vi "Main.vi"(10 "VISA resource name":refnum<visa-resource-name>="COM11", 11 "Module Admin":refnum<class "Delacor_lib_QMH_Module Admin.lvclass">) -> ()   [LabVIEW 2018, in "MB switches Module.lvlib"]
doc: "This template is based off of the Queued Message Handler design pattern and the Queued Message Handler project template that ships with LabVIEW.\n\nThe main difference is that the queue is private to this module and communication between modules is performed via Broadcast and Request events.\n\nRequest events are wrapped in public API methods and are handled in the Event Handling Loop (EHL) of this VI. Any module can register for Broadcast events sent by this module. The EHL generates messages based on user interface actions.\n\nThe Message Handling Loop (MHL) processes messages generated by the EHL, or by other messages. The messages are string values, so new messages can be added easily to the Message Cases case structure in the MHL. Each message cluster can also provide an optional value for Message Data, which is a variant that can be converted to whatever message-specific data is required.\n_____\nBased on DQMH Project Template 6.0.0.91."
uses:
  MB switches Module.lvlib
  <vilib>/Delacor/Delacor QMH/Libraries/Module Admin_class/Delacor_lib_QMH_Module Admin.lvclass
  Module Data--cluster.ctl
  <vilib>/NI/Modbus Library/API/Master/Modbus Master.lvclass
  Do Something Else and Wait for Reply Argument--cluster.ctl
  Do Something Else and Wait (Reply Payload)--cluster.ctl
  <vilib>/Delacor/Delacor QMH/Libraries/Message Queue_class/Delacor_lib_QMH_Message Queue.lvclass/Delacor_lib_QMH_Message Queue.ctl
  Stop Argument--cluster.ctl
  <vilib>/Delacor/Delacor QMH/Libraries/Module Admin_class/Delacor_lib_QMH_Module Admin.lvclass/Delacor_lib_QMH_Module Admin.ctl
  inst.Counter Argument--cluster.ctl
  inst.Counter (Reply Payload)--cluster.ctl
  inst.Optos Argument--cluster.ctl
  inst.Optos (Reply Payload)--cluster.ctl
  mux10-1_chan0 Argument--cluster.ctl
  mux6-1_chan0 Argument--cluster.ctl
  inst.Open Argument--cluster.ctl
  inst.Close Argument--cluster.ctl
  DMM I 0.5_10 Argument--cluster.ctl
  mux10-1_chan1 Argument--cluster.ctl
  mux10-1_chan2 Argument--cluster.ctl
  mux10-1_chan3 Argument--cluster.ctl
  mux10-1_chan4 Argument--cluster.ctl
  mux10-1_chan5 Argument--cluster.ctl
  mux10-1_chan6 Argument--cluster.ctl
  mux10-1_chan7 Argument--cluster.ctl
  mux10-1_chan8 Argument--cluster.ctl
  mux10-1_chan9 Argument--cluster.ctl
  mux10-1_chan10 Argument--cluster.ctl
  mux6-1_chan1_1 Argument--cluster.ctl
  mux6-1_chan1_2 Argument--cluster.ctl
  mux6-1_chan2_1 Argument--cluster.ctl
  mux6-1_chan2_2 Argument--cluster.ctl
  mux6-1_chan3_1 Argument--cluster.ctl
  mux6-1_chan3_2 Argument--cluster.ctl
  mux6-1_chan4_1 Argument--cluster.ctl
  mux6-1_chan4_2 Argument--cluster.ctl
  mux6-1_chan5_1 Argument--cluster.ctl
  mux6-1_chan5_2 Argument--cluster.ctl
  mux6-1_chan6_1 Argument--cluster.ctl
  mux6-1_chan6_2 Argument--cluster.ctl
  <vilib>/Utility/miscctls.llb/LVPointTypeDef.ctl
  <vilib>/Delacor/Delacor QMH/Libraries/Message Queue_class/Delacor_lib_QMH_Enqueue Message (Single).vi
  <vilib>/Delacor/Delacor QMH/Libraries/Module Admin_class/Delacor_lib_QMH_Get External Launch.vi
  <vilib>/Utility/error.llb/Error Cluster From Error Code.vi
  <vilib>/ErrorRing/Error Ring.xnode
  <vilib>/Delacor/Delacor QMH/Libraries/Message Queue_class/Delacor_lib_QMH_Message Queue.lvclass
  Instrument Drivers/LV_driver_MBrelay/MB Relay.lvlib
  Instrument Drivers/LV_driver_MBrelay/type defs/FGV enum.ctl
panel:
  out "error out":errorcluster
  out "Status":string
  in  "Simulate MHL Error":bool
  in  "Simulate EHL Error":bool
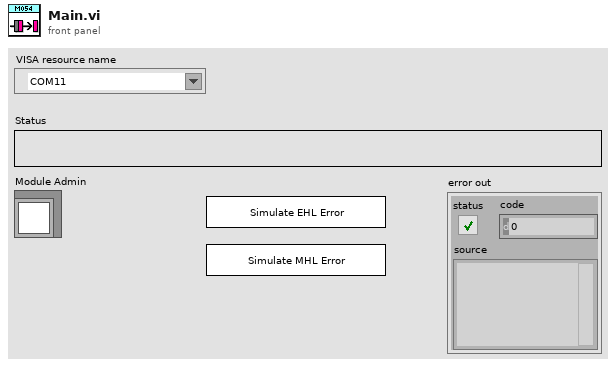
[diagram p1: front panel]
types:
  T1 = typedef "MB switches Module.lvlib/Request Events--cluster.ctl" = cluster{"Stop Module":refnum<user-event>, "Do Something Else and Wait for Reply":refnum<user-event>, "Show Panel":refnum<user-event>, "Hide Panel":refnum<user-event>, "Get Module Execution Status":refnum<user-event>, "Show Diagram":refnum<user-event>, "inst.Counter":refnum<user-event>, "inst.Open":refnum<user-event>, "inst.Close":refnum<user-event>, "inst.Optos":refnum<user-event>, "mux10-1_chan0":refnum<user-event>, "mux6-1_chan0":refnum<user-event>, "DMM I 0.5_10":refnum<user-event>, "mux10-1_chan1":refnum<user-event>, "mux10-1_chan2":refnum<user-event>, "mux10-1_chan3":refnum<user-event>, "mux10-1_chan4":refnum<user-event>, "mux10-1_chan5":refnum<user-event>, "mux10-1_chan6":refnum<user-event>, "mux10-1_chan7":refnum<user-event>, "mux10-1_chan8":refnum<user-event>, "mux10-1_chan9":refnum<user-event>, "mux10-1_chan10":refnum<user-event>, "mux6-1_chan1_1":refnum<user-event>, "mux6-1_chan1_2":refnum<user-event>, "mux6-1_chan2_1":refnum<user-event>, "mux6-1_chan2_2":refnum<user-event>, "mux6-1_chan3_1":refnum<user-event>, "mux6-1_chan3_2":refnum<user-event>, "mux6-1_chan4_1":refnum<user-event>, "mux6-1_chan4_2":refnum<user-event>, "mux6-1_chan5_1":refnum<user-event>, "mux6-1_chan5_2":refnum<user-event>, "mux6-1_chan6_1":refnum<user-event>, "mux6-1_chan6_2":refnum<user-event>}
  T2 = typedef "MB switches Module.lvlib/Module Data--cluster.ctl" = cluster{"Status":string, "Modbus Master ref":refnum<class "Modbus Master.lvclass">, "VISA resource name":refnum<visa-resource-name>}
  T3 = typedef "MB switches Module.lvlib/Do Something Else and Wait for Reply Argument--cluster.ctl" = cluster{"Do Something Else Msg":string, "X":dbl, "Wait Notifier":refnum<notifier>, "wait for reply":bool}
  T4 = enum32{"invalid lock state", "Not Locked", "Locked (No Password)", "Password-protected"}
  T5 = typedef "MB switches Module.lvlib/Stop Argument--cluster.ctl" = cluster{"Origin":string, "Exit via Stop Module Req?":bool, "Wait for Module to stop?":bool}
  T6 = typedef "MB switches Module.lvlib/inst.Counter Argument--cluster.ctl" = cluster{"Wait Notifier":refnum<notifier>, "wait for reply":bool}
  T7 = typedef "MB switches Module.lvlib/inst.Optos Argument--cluster.ctl" = cluster{"Wait Notifier":refnum<notifier>, "wait for reply":bool}
  T8 = typedef "MB switches Module.lvlib/mux10-1_chan0 Argument--cluster.ctl" = cluster{"mux10_1(x6)_encode":enum16{"mux10_1_channel0", "mux10_1_channel1", "mux10_1_channel2", "mux10_1_channel3", "mux10_1_channel4", "mux10_1_channel5", "mux10_1_channel6", "mux10_1_channel7", "mux10_1_channel8", "mux10_1_channel9", "mux10_1_channel10"}}
  T9 = typedef "MB switches Module.lvlib/mux6-1_chan0 Argument--cluster.ctl" = cluster{"mux6_1(3wires)_encode":enum16{"mux6-1_channel0", "mux6_1_channel1_0", "mux6_1_channel1_1", "mux6-1_channel1_2", "mux6_1_channel1_3", "mux6_1_channel2_0", "mux6_1_channel2_1", "mux6_1_channel2_2", "mux6_1_channel2_3", "mux6_1_channel3_0", "mux6_1_channel3_1", "mux6_1_channel3_2", "mux6_1_channel3_3", "mux6_1_channel4_0", "mux6_1_channel4_1", "mux6_1_channel4_2", "mux6_1_channel4_3", "mux6_1_channel5_0", "mux6_1_channel5_1", "mux6_1_channel5_2", "mux6_1_channel5_3", "mux6_1_channel6_0", "mux6_1_channel6_1", "mux6_1_channel6_2", "mux6_1_channel6_3"}}
  T10 = typedef "MB switches Module.lvlib/DMM I 0.5_10 Argument--cluster.ctl" = cluster{"mux2-1(DMM I) encode":enum16{"DMM I (0.5)", "DMM I (12)"}}
  T11 = typedef "MB switches Module.lvlib/mux10-1_chan1 Argument--cluster.ctl" = cluster{"Boolean":bool}
  T12 = typedef "MB switches Module.lvlib/mux10-1_chan2 Argument--cluster.ctl" = cluster{"Boolean":bool}
  T13 = typedef "MB switches Module.lvlib/mux10-1_chan3 Argument--cluster.ctl" = cluster{"Boolean":bool}
  T14 = typedef "MB switches Module.lvlib/mux10-1_chan4 Argument--cluster.ctl" = cluster{"Boolean":bool}
  T15 = typedef "MB switches Module.lvlib/mux10-1_chan5 Argument--cluster.ctl" = cluster{"Boolean":bool}
  T16 = typedef "MB switches Module.lvlib/mux10-1_chan6 Argument--cluster.ctl" = cluster{"Boolean":bool}
  T17 = typedef "MB switches Module.lvlib/mux10-1_chan7 Argument--cluster.ctl" = cluster{"Boolean":bool}
  T18 = typedef "MB switches Module.lvlib/mux10-1_chan8 Argument--cluster.ctl" = cluster{"Boolean":bool}
  T19 = typedef "MB switches Module.lvlib/mux10-1_chan9 Argument--cluster.ctl" = cluster{"Boolean":bool}
  T20 = typedef "MB switches Module.lvlib/mux10-1_chan10 Argument--cluster.ctl" = cluster{"Boolean":bool}
  T21 = typedef "MB switches Module.lvlib/mux6-1_chan1_1 Argument--cluster.ctl" = cluster{"Boolean":bool}
  T22 = typedef "MB switches Module.lvlib/mux6-1_chan1_2 Argument--cluster.ctl" = cluster{"Boolean":bool}
  T23 = typedef "MB switches Module.lvlib/mux6-1_chan2_1 Argument--cluster.ctl" = cluster{"Boolean":bool}
  T24 = typedef "MB switches Module.lvlib/mux6-1_chan2_2 Argument--cluster.ctl" = cluster{"Boolean":bool}
  T25 = typedef "MB switches Module.lvlib/mux6-1_chan3_1 Argument--cluster.ctl" = cluster{"Boolean":bool}
  T26 = typedef "MB switches Module.lvlib/mux6-1_chan3_2 Argument--cluster.ctl" = cluster{"Boolean":bool}
  T27 = typedef "MB switches Module.lvlib/mux6-1_chan4_1 Argument--cluster.ctl" = cluster{"Boolean":bool}
  T28 = typedef "MB switches Module.lvlib/mux6-1_chan4_2 Argument--cluster.ctl" = cluster{"Boolean":bool}
  T29 = typedef "MB switches Module.lvlib/mux6-1_chan5_1 Argument--cluster.ctl" = cluster{"Boolean":bool}
  T30 = typedef "MB switches Module.lvlib/mux6-1_chan5_2 Argument--cluster.ctl" = cluster{"Boolean":bool}
  T31 = typedef "MB switches Module.lvlib/mux6-1_chan6_1 Argument--cluster.ctl" = cluster{"Boolean":bool}
  T32 = typedef "MB switches Module.lvlib/mux6-1_chan6_2 Argument--cluster.ctl" = cluster{"Boolean":bool}
  T33 = typedef "LVPointTypeDef.ctl" = cluster{"Horizontal":i16, "Vertical":i16}
  T34 = enum32{"Invalid", "Standard", "Closed", "Hidden", "Minimized", "Maximized"}
  T35 = typedef "MB switches Module.lvlib/Do Something Else and Wait (Reply Payload)--cluster.ctl" = cluster{"Value":dbl, "error":errorcluster}
  T36 = typedef "MB switches Module.lvlib/inst.Open Argument--cluster.ctl" = cluster{"VISA resource name":refnum<visa-resource-name>}
  T37 = typedef "MB switches Module.lvlib/inst.Close Argument--cluster.ctl" = cluster{"Boolean":bool}
  T38 = typedef "MB Relay.lvlib/FGV enum.ctl" = enum16{"Write", "Init FGV", "Read", "All OFF", "All ON"}
  T39 = typedef "MB switches Module.lvlib/inst.Counter (Reply Payload)--cluster.ctl" = cluster{"counter":u16, "inst.Counter_error":errorcluster}
  T40 = typedef "MB switches Module.lvlib/inst.Optos (Reply Payload)--cluster.ctl" = cluster{"Optos":bool[], "inst.Optos_error":errorcluster}
  T41 = enum16{"mux10_1_channel0", "mux10_1_channel1", "mux10_1_channel2", "mux10_1_channel3", "mux10_1_channel4", "mux10_1_channel5", "mux10_1_channel6", "mux10_1_channel7", "mux10_1_channel8", "mux10_1_channel9", "mux10_1_channel10"}
  T42 = enum16{"mux6-1_channel0", "mux6_1_channel1_0", "mux6_1_channel1_1", "mux6-1_channel1_2", "mux6_1_channel1_3", "mux6_1_channel2_0", "mux6_1_channel2_1", "mux6_1_channel2_2", "mux6_1_channel2_3", "mux6_1_channel3_0", "mux6_1_channel3_1", "mux6_1_channel3_2", "mux6_1_channel3_3", "mux6_1_channel4_0", "mux6_1_channel4_1", "mux6_1_channel4_2", "mux6_1_channel4_3", "mux6_1_channel5_0", "mux6_1_channel5_1", "mux6_1_channel5_2", "mux6_1_channel5_3", "mux6_1_channel6_0", "mux6_1_channel6_1", "mux6_1_channel6_2", "mux6_1_channel6_3"}
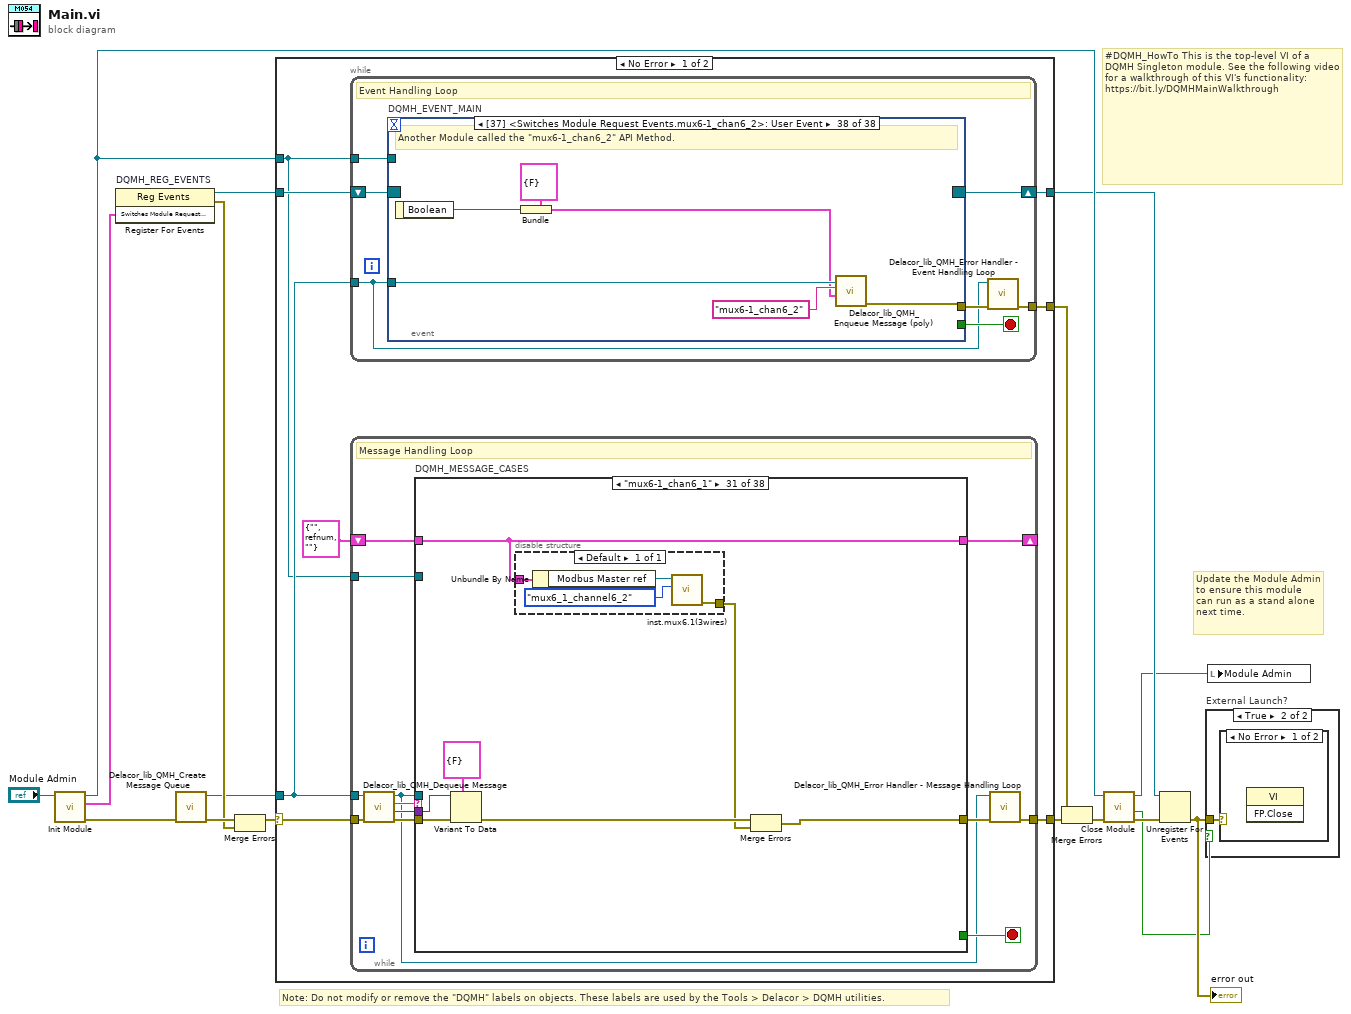
[diagram p0: block diagram]
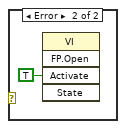
[diagram p3: hidden frame]
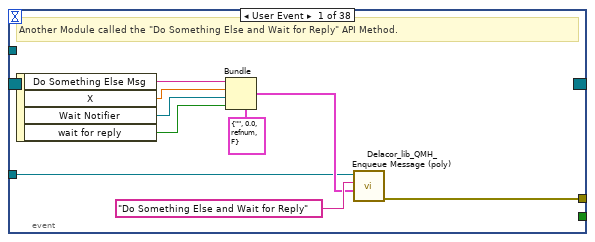
[diagram p4: hidden frame]
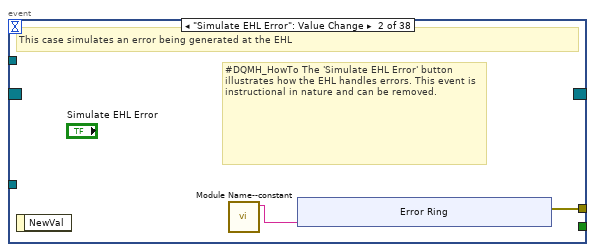
[diagram p5: hidden frame]
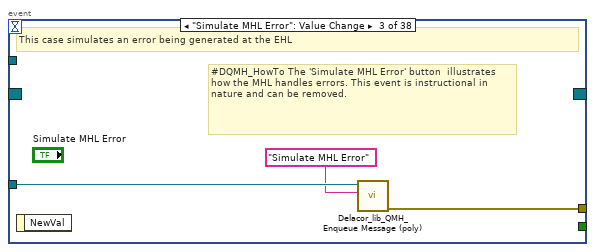
[diagram p6: hidden frame]
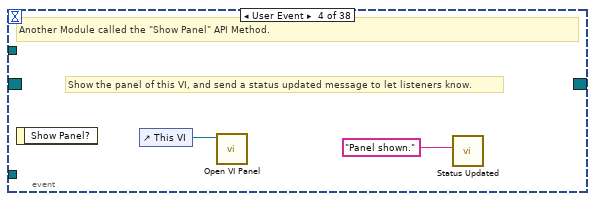
[diagram p7: hidden frame]
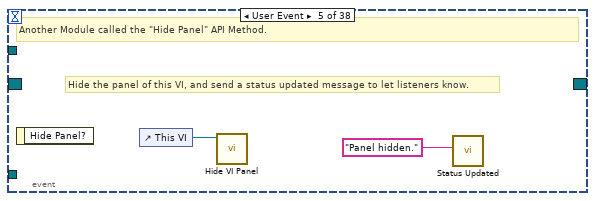
[diagram p8: hidden frame]
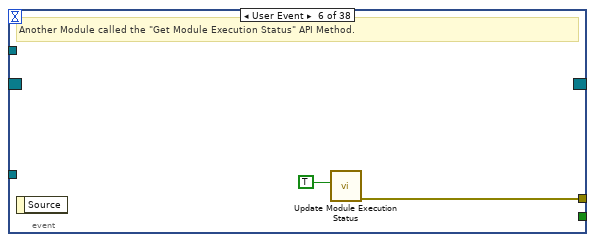
[diagram p9: hidden frame]
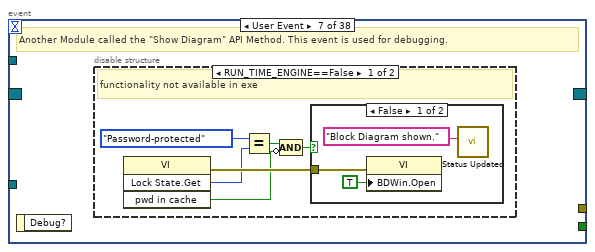
[diagram p10: hidden frame]
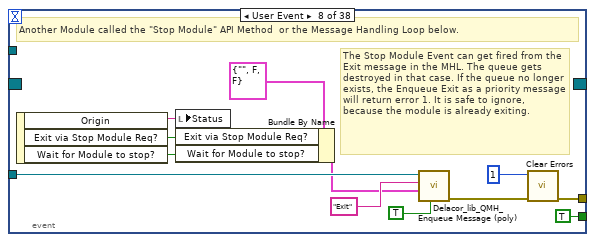
[diagram p13: hidden frame]
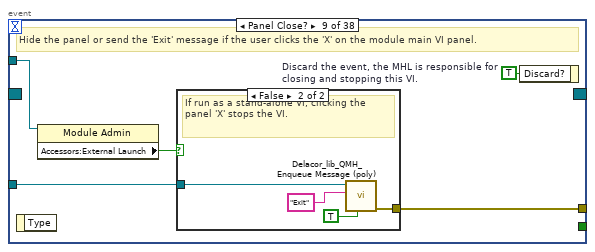
[diagram p14: hidden frame]
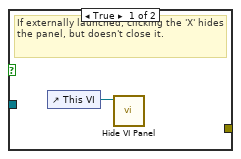
[diagram p15: hidden frame]
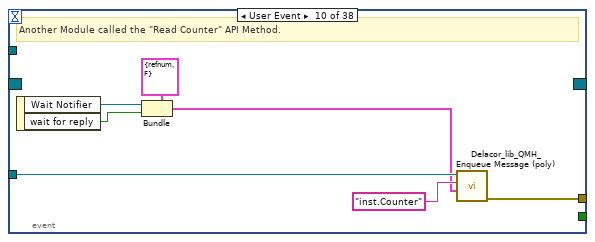
[diagram p16: hidden frame]
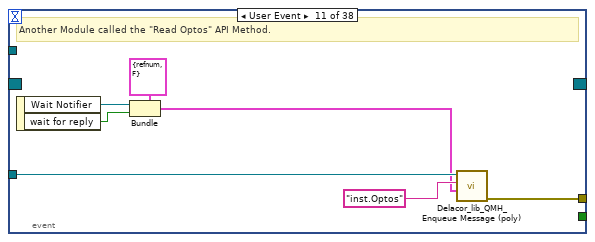
[diagram p17: hidden frame]
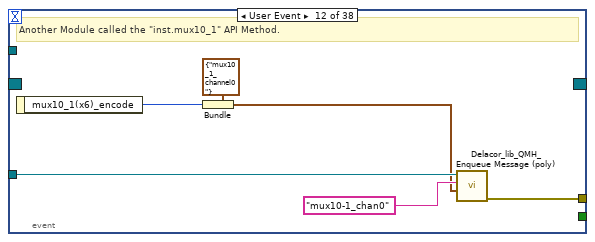
[diagram p18: hidden frame]
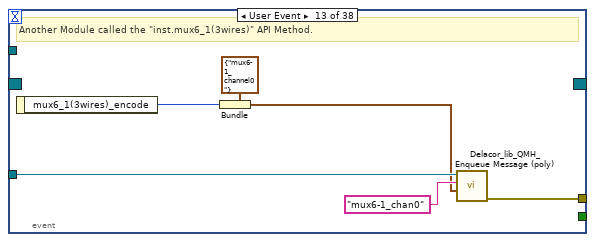
[diagram p19: hidden frame]
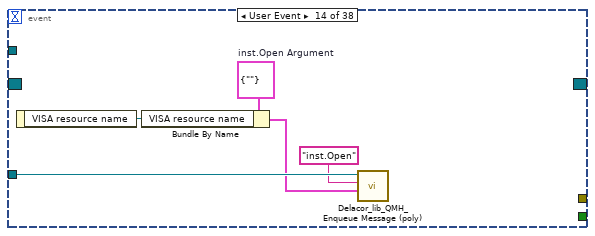
[diagram p20: hidden frame]
diagram:
  # "#DQMH_HowTo This is the top-level VI of a DQMH Singleton module. See the following video for a walkthrough of this VI's functionality: https://bit.ly/DQMHMainWalkthrough"
  # "Note: Do not modify or remove the \"DQMH\" labels on objects. These labels are used by the Tools > Delacor > DQMH utilities."
  # "Update the Module Admin to ensure this module can run as a stand alone next time."
  n1 = call "Init Module.vi"("Singleton Module Admin in"="Module Admin") -> ("error out"=w16:errorcluster, "Switches Module Request Events"=w2:T1, "Singleton Module Admin out"=w8:refnum<class "Delacor_lib_QMH_Module Admin.lvclass">)  [unwired: 8 in]
  n2 = register-events "DQMH_REG_EVENTS"(w2) -> (reference out=w1:refnum<event-registration>, error out=w9:errorcluster)  [unwired: 2 in]
  n3 = call <vilib>:"Delacor_lib_QMH_Create Message Queue.vi"("error in"=w16) -> ("error out"=w11:errorcluster, "Message Queue"=w6:refnum<class "Delacor_lib_QMH_Message Queue.lvclass">)  [unwired: 9 in]
  n4 = Merge Errors(w11, w9) -> (w10:errorcluster)
  n5 = case shown="No Error" w10 {
    selector: w10 -> [w23 w762]
    tunnel: [w25 w761] -> w17
    tunnel: [w22 w767] -> w7
    tunnel: w1 -> [w20 w767]
    tunnel: w6 -> [w19 w760]
    tunnel: [w24 _] -> w14
    tunnel: w8 -> [w18 w763]
    frame No Error {
      n6 = while {
        tunnel: w19 -> [w26]
        shift-right: [w29] -> w22
        shift-left: w20 -> [w30]
        tunnel: [w31] -> w24
        tunnel: w18 -> [w27]
        stop <- w28 stop-if-true
        # "Event Handling Loop"
        n7 = event "DQMH_EVENT_MAIN" shown="[37] <Switches Module Request Events.mux6-1_chan6_2>: User Event" {
          selector: w30 -> [_ _ _ _ _ _ _ _ _ _ _ _ _ _ _ _ _ _ _ _ _ _ _ _ _ _ _ _ _ _ _ _ _ _ _ _ _ _]
          dyn-events: [_ _ _ _ _ _ _ _ _ _ _ _ _ _ _ _ _ _ _ _ _ _ _ _ _ _ _ _ _ _ _ _ _ _ _ _ _ _] -> w29
          timeout: _ -> [_ _ _ _ _ _ _ _ _ _ _ _ _ _ _ _ _ _ _ _ _ _ _ _ _ _ _ _ _ _ _ _ _ _ _ _ _ _]
          tunnel: [_ _ _ _ _ _ _ TRUE ("Discard?") _ _ _ _ _ _ _ _ _ _ _ _ _ _ _ _ _ _ _ _ _ _ _ _ _ _ _ _ _ _] -> w28
          tunnel: w26 -> [w34 _ w52 _ _ _ _ w76 w83 w97 w104 w110 w116 w121 w123 w132 w138 w144 w150 w156 w162 w168 w174 w180 w186 w192 w198 w204 w210 w216 w222 w228 w234 w240 w246 w252 w258 w264]
          tunnel: [w41 w43 w53 _ _ w59 _ w79 w85 w91 w98 w105 w111 _ _ w127 w133 w139 w145 w151 w157 w163 w169 w175 w181 w187 w193 w199 w205 w211 w217 w223 w229 w235 w241 w247 w253 w259] -> w32
          tunnel: w27 -> [_ _ _ _ _ _ _ _ w82 _ _ _ _ _ _ _ _ _ _ _ _ _ _ _ _ _ _ _ _ _ _ _ _ _ _ _ _ _]
          event User Event {
            # "Another Module called the \"Do Something Else and Wait for Reply\" API Method."
            n8 = event-data() -> ("Do Something Else Msg"=w37:string, "X"=w36:dbl, "Wait Notifier"=w35:refnum<notifier>, "wait for reply"=w33:bool)  [unwired: 1 in]
            n9 = Bundle(cluster=T3 {"Do Something Else Msg"="", "X"=0.0, "Wait Notifier"=refnum, "wait for reply"=FALSE} ("Do Something Else and Wait for Reply Argument"), "Do Something Else Msg"=w37, "X"=w36, "Wait Notifier"=w35, "wait for reply"=w33) -> (w38:T3)
            n10 = call-poly <vilib>:"Delacor_lib_QMH_Enqueue Message (poly).vi"("Message Data"=w38, "Message"="Do Something Else and Wait for Reply", "Message Queue in"=w34) -> ("error out"=w41:errorcluster)  [unwired: 7 in, 1 out]
          }
          event "Simulate EHL Error": Value Change {
            # "#DQMH_HowTo The 'Simulate EHL Error' button  illustrates how the EHL handles errors. This event is instructional in nature and can be removed."
            # "This case simulates an error being generated at the EHL"
            n11 = event-data() -> ()  [unwired: 1 in, 1 out]
            n12 = call "Module Name--constant.vi"() -> ("Module Name"=w42:string)  [unwired: 11 in]
            n13 = xnode "Error Ring"("parameter 0"=w42) -> ("error out"=w43:errorcluster)
          }
          event "Simulate MHL Error": Value Change {
            # "#DQMH_HowTo The 'Simulate MHL Error' button  illustrates how the MHL handles errors. This event is instructional in nature and can be removed."
            # "This case simulates an error being generated at the EHL"
            n14 = event-data() -> ()  [unwired: 1 in, 1 out]
            n15 = call-poly <vilib>:"Delacor_lib_QMH_Enqueue Message (poly).vi"("Message"="Simulate MHL Error", "Message Queue in"=w52) -> ("error out"=w53:errorcluster)  [unwired: 8 in, 1 out]
          }
          event User Event {
            # "Show the panel of this VI, and send a status updated message to let listeners know."
            # "Another Module called the \"Show Panel\" API Method."
            n16 = event-data() -> ()  [unwired: 1 in, 1 out]
            n17 = control-ref of="This VI"() -> (w55:refnum<vi>)
            n18 = call "Open VI Panel.vi"("VI"=w55) -> ()  [unwired: 10 in, 1 out]
            n19 = call "Status Updated.vi"("Status"="Panel shown." ("format string")) -> ()  [unwired: 10 in, 1 out]
          }
          event User Event {
            # "Hide the panel of this VI, and send a status updated message to let listeners know."
            # "Another Module called the \"Hide Panel\" API Method."
            n20 = event-data() -> ()  [unwired: 1 in, 1 out]
            n21 = control-ref of="This VI"() -> (w57:refnum<vi>)
            n22 = call "Hide VI Panel.vi"("VI"=w57) -> ()  [unwired: 10 in, 1 out]
            n23 = call "Status Updated.vi"("Status"="Panel hidden." ("format string")) -> ()  [unwired: 10 in, 1 out]
          }
          event User Event {
            # "Another Module called the \"Get Module Execution Status\" API Method."
            n24 = event-data() -> ()  [unwired: 1 in, 1 out]
            n25 = call "Update Module Execution Status.vi"("Running?"=TRUE) -> ("error out"=w59:errorcluster)  [unwired: 10 in]
          }
          event User Event {
            # "Another Module called the \"Show Diagram\" API Method. This event is used for debugging."
            n26 = event-data() -> ()  [unwired: 1 in, 1 out]
            n27 = disable-structure shown="RUN_TIME_ENGINE==False" {
              frame condition #0 (active) {
                # "functionality not available in exe"
                n28 = invoke class="VI" method="Lock State.Get"() -> (error out=w65:errorcluster, "Get Lock State"=w64:T4, "pwd in cache"=w61:bool)  [unwired: 4 in, 1 out]
                n29 = Equal?(x=T4."Password-protected", y=w64) -> (x = y?=w62:bool)
                n30 = Compound Arithmetic op=AND(w62, invert w61) -> (w60:bool)
                n31 = case shown="False" w60 {
                  tunnel: w65 -> [w68 _]
                  frame False {
                    n32 = property class="VI"(error in=w68, "BDWin.Open"=TRUE ("Block Diagram Window:Open")) -> ()  [unwired: 1 in, 2 out]
                    n33 = call "Status Updated.vi"("Status"="Block Diagram shown." ("format string")) -> ()  [unwired: 10 in, 1 out]
                  }
                  frame True {
                    # "Password-protected VI, and the password is not in the cache. Do not show the diagram."
                  }
                }
              }
              frame condition #1 {
              }
            }
          }
          event User Event {
            # "The Stop Module Event can get fired from the Exit message in the MHL. The queue gets destroyed in that case. If the queue no longer exists, the Enqueue Exit as a priority message will return error 1. It is safe to ignore, because the module is already exiting."
            # "Another Module called the \"Stop Module\" API Method  or the Message Handling Loop below."
            n34 = event-data() -> ("Origin"=w75:string, "Exit via Stop Module Req?"=w71:bool, "Wait for Module to stop?"=w70:bool)  [unwired: 1 in]
            n35 = local write "Status"(w75) -> ()
            n36 = Bundle By Name(cluster=T5 {"Origin"="", "Exit via Stop Module Req?"=FALSE, "Wait for Module to stop?"=FALSE} ("Stop Argument"), "Exit via Stop Module Req?"=w71, "Wait for Module to stop?"=w70) -> (w69:T5)
            n37 = call-poly <vilib>:"Delacor_lib_QMH_Enqueue Message (poly).vi"("Priority Message? (F)"=TRUE, "Message Data"=w69, "Message"="Exit", "Message Queue in"=w76) -> ("error out"=w80:errorcluster)  [unwired: 6 in, 1 out]
            n38 = call <vilib>:"Clear Errors.vi"("error in (no error)"=w80, "specific error code to clear (0: all)"=1) -> ("error out"=w79:errorcluster)  [unwired: 4 in, 1 out]
          }
          event Panel Close? {
            w84 = TRUE  # Discard the event, the MHL is responsible for closing and stopping this VI.
            # "Hide the panel or send the 'Exit' message if the user clicks the 'X' on the module main VI panel."
            n39 = event-data() -> ()  [unwired: 1 in, 1 out]
            n40 = property class="Module Admin"(reference=w82) -> ("Accessors:External Launch"=w81:bool)  [unwired: 1 in, 2 out]
            n41 = case shown="False" w81 {
              tunnel: w83 -> [_ w89]
              tunnel: [_ w90] -> w85
              frame True {
                # "If externally launched, clicking the 'X' hides the panel, but doesn't close it."
                n42 = control-ref of="This VI"() -> (w86:refnum<vi>)
                n43 = call "Hide VI Panel.vi"("VI"=w86) -> ()  [unwired: 10 in, 1 out]
              }
              frame False {
                # "If run as a stand-alone VI, clicking the panel 'X' stops the VI."
                n44 = call-poly <vilib>:"Delacor_lib_QMH_Enqueue Message (poly).vi"("Priority Message? (F)"=TRUE, "Message"="Exit", "Message Queue in"=w89) -> ("error out"=w90:errorcluster)  [unwired: 7 in, 1 out]
              }
            }
            n45 = event-data("Discard?"=w84) -> ()  [unwired: 1 in, 1 out]
          }
          event User Event {
            # "Another Module called the \"Read Counter\" API Method."
            n46 = event-data() -> ("Wait Notifier"=w93:refnum<notifier>, "wait for reply"=w92:bool)  [unwired: 1 in]
            n47 = Bundle(cluster=T6 {"Wait Notifier"=refnum, "wait for reply"=FALSE} ("Read Counter Argument"), "Wait Notifier"=w93, "wait for reply"=w92) -> (w94:T6)
            n48 = call-poly <vilib>:"Delacor_lib_QMH_Enqueue Message (poly).vi"("Message Data"=w94, "Message"="inst.Counter", "Message Queue in"=w97) -> ("error out"=w91:errorcluster)  [unwired: 7 in, 1 out]
          }
          event User Event {
            # "Another Module called the \"Read Optos\" API Method."
            n49 = event-data() -> ("Wait Notifier"=w100:refnum<notifier>, "wait for reply"=w99:bool)  [unwired: 1 in]
            n50 = Bundle(cluster=T7 {"Wait Notifier"=refnum, "wait for reply"=FALSE} ("Read Optos Argument"), "Wait Notifier"=w100, "wait for reply"=w99) -> (w101:T7)
            n51 = call-poly <vilib>:"Delacor_lib_QMH_Enqueue Message (poly).vi"("Message Data"=w101, "Message"="inst.Optos", "Message Queue in"=w104) -> ("error out"=w98:errorcluster)  [unwired: 7 in, 1 out]
          }
          event User Event {
            # "Another Module called the \"inst.mux10_1\" API Method."
            n52 = event-data() -> ("mux10_1(x6)_encode"=w106:T41)  [unwired: 1 in]
            n53 = Bundle(cluster=T8 {"mux10_1(x6)_encode"=enum."mux10_1_channel0"} ("inst.mux10_1 Argument"), "mux10_1(x6)_encode"=w106) -> (w107:T8)
            n54 = call-poly <vilib>:"Delacor_lib_QMH_Enqueue Message (poly).vi"("Message Data"=w107, "Message"="mux10-1_chan0", "Message Queue in"=w110) -> ("error out"=w105:errorcluster)  [unwired: 7 in, 1 out]
          }
          event User Event {
            # "Another Module called the \"inst.mux6_1(3wires)\" API Method."
            n55 = event-data() -> ("mux6_1(3wires)_encode"=w112:T42)  [unwired: 1 in]
            n56 = Bundle(cluster=T9 {"mux6_1(3wires)_encode"=enum."mux6-1_channel0"} ("inst.mux6_1(3wires) Argument"), "mux6_1(3wires)_encode"=w112) -> (w113:T9)
            n57 = call-poly <vilib>:"Delacor_lib_QMH_Enqueue Message (poly).vi"("Message Data"=w113, "Message"="mux6-1_chan0", "Message Queue in"=w116) -> ("error out"=w111:errorcluster)  [unwired: 7 in, 1 out]
          }
          event User Event {
            w119 = T36 {"VISA resource name"=""}  # inst.Open Argument
            n58 = event-data() -> ("VISA resource name"=w118:refnum<visa-resource-name>)  [unwired: 1 in]
            n59 = Bundle By Name(cluster=w119, "VISA resource name"=w118) -> (w117:T36)
            n60 = call-poly <vilib>:"Delacor_lib_QMH_Enqueue Message (poly).vi"("Message Data"=w117, "Message"="inst.Open", "Message Queue in"=w121) -> ()  [unwired: 7 in, 2 out]
          }
          event User Event {
            w126 = T37 {"Boolean"=FALSE}  # inst.Close Argument
            n61 = event-data() -> ("Boolean"=w125:bool)  [unwired: 1 in]
            n62 = Bundle By Name(cluster=w126, "Boolean"=w125) -> (w124:T37)
            n63 = call-poly <vilib>:"Delacor_lib_QMH_Enqueue Message (poly).vi"("Message Data"=w124, "Message"="inst.Close", "Message Queue in"=w123) -> ()  [unwired: 7 in, 2 out]
          }
          event User Event {
            # "Another Module called the \"DMM I 0.5_10\" API Method."
            n64 = event-data() -> ("mux2-1(DMM I) encode"=w128:enum16{"DMM I (0.5)", "DMM I (12)"})  [unwired: 1 in]
            n65 = Bundle(cluster=T10 {"mux2-1(DMM I) encode"=enum."DMM I (0.5)"} ("DMM I 0.5_10 Argument"), "mux2-1(DMM I) encode"=w128) -> (w129:T10)
            n66 = call-poly <vilib>:"Delacor_lib_QMH_Enqueue Message (poly).vi"("Message Data"=w129, "Message"="DMM I 0.5_10", "Message Queue in"=w132) -> ("error out"=w127:errorcluster)  [unwired: 7 in, 1 out]
          }
          event User Event {
            # "Another Module called the \"mux10-1_chan1\" API Method."
            n67 = event-data() -> ("Boolean"=w134:bool)  [unwired: 1 in]
            n68 = Bundle(cluster=T11 {"Boolean"=FALSE} ("mux10-1_chan1 Argument"), "Boolean"=w134) -> (w135:T11)
            n69 = call-poly <vilib>:"Delacor_lib_QMH_Enqueue Message (poly).vi"("Message Data"=w135, "Message"="mux10-1_chan1", "Message Queue in"=w138) -> ("error out"=w133:errorcluster)  [unwired: 7 in, 1 out]
          }
          event User Event {
            # "Another Module called the \"mux10-1_chan2\" API Method."
            n70 = event-data() -> ("Boolean"=w140:bool)  [unwired: 1 in]
            n71 = Bundle(cluster=T12 {"Boolean"=FALSE} ("mux10-1_chan2 Argument"), "Boolean"=w140) -> (w141:T12)
            n72 = call-poly <vilib>:"Delacor_lib_QMH_Enqueue Message (poly).vi"("Message Data"=w141, "Message"="mux10-1_chan2", "Message Queue in"=w144) -> ("error out"=w139:errorcluster)  [unwired: 7 in, 1 out]
          }
          event User Event {
            # "Another Module called the \"mux10-1_chan3\" API Method."
            n73 = event-data() -> ("Boolean"=w146:bool)  [unwired: 1 in]
            n74 = Bundle(cluster=T13 {"Boolean"=FALSE} ("mux10-1_chan3 Argument"), "Boolean"=w146) -> (w147:T13)
            n75 = call-poly <vilib>:"Delacor_lib_QMH_Enqueue Message (poly).vi"("Message Data"=w147, "Message"="mux10-1_chan3", "Message Queue in"=w150) -> ("error out"=w145:errorcluster)  [unwired: 7 in, 1 out]
          }
          event User Event {
            # "Another Module called the \"mux10-1_chan4\" API Method."
            n76 = event-data() -> ("Boolean"=w152:bool)  [unwired: 1 in]
            n77 = Bundle(cluster=T14 {"Boolean"=FALSE} ("mux10-1_chan4 Argument"), "Boolean"=w152) -> (w153:T14)
            n78 = call-poly <vilib>:"Delacor_lib_QMH_Enqueue Message (poly).vi"("Message Data"=w153, "Message"="mux10-1_chan4", "Message Queue in"=w156) -> ("error out"=w151:errorcluster)  [unwired: 7 in, 1 out]
          }
          event User Event {
            # "Another Module called the \"mux10-1_chan5\" API Method."
            n79 = event-data() -> ("Boolean"=w158:bool)  [unwired: 1 in]
            n80 = Bundle(cluster=T15 {"Boolean"=FALSE} ("mux10-1_chan5 Argument"), "Boolean"=w158) -> (w159:T15)
            n81 = call-poly <vilib>:"Delacor_lib_QMH_Enqueue Message (poly).vi"("Message Data"=w159, "Message"="mux10-1_chan5", "Message Queue in"=w162) -> ("error out"=w157:errorcluster)  [unwired: 7 in, 1 out]
          }
          event User Event {
            # "Another Module called the \"mux10-1_chan6\" API Method."
            n82 = event-data() -> ("Boolean"=w164:bool)  [unwired: 1 in]
            n83 = Bundle(cluster=T16 {"Boolean"=FALSE} ("mux10-1_chan6 Argument"), "Boolean"=w164) -> (w165:T16)
            n84 = call-poly <vilib>:"Delacor_lib_QMH_Enqueue Message (poly).vi"("Message Data"=w165, "Message"="mux10-1_chan6", "Message Queue in"=w168) -> ("error out"=w163:errorcluster)  [unwired: 7 in, 1 out]
          }
          event User Event {
            # "Another Module called the \"mux10-1_chan7\" API Method."
            n85 = event-data() -> ("Boolean"=w170:bool)  [unwired: 1 in]
            n86 = Bundle(cluster=T17 {"Boolean"=FALSE} ("mux10-1_chan7 Argument"), "Boolean"=w170) -> (w171:T17)
            n87 = call-poly <vilib>:"Delacor_lib_QMH_Enqueue Message (poly).vi"("Message Data"=w171, "Message"="mux10-1_chan7", "Message Queue in"=w174) -> ("error out"=w169:errorcluster)  [unwired: 7 in, 1 out]
          }
          event User Event {
            # "Another Module called the \"mux10-1_chan8\" API Method."
            n88 = event-data() -> ("Boolean"=w176:bool)  [unwired: 1 in]
            n89 = Bundle(cluster=T18 {"Boolean"=FALSE} ("mux10-1_chan8 Argument"), "Boolean"=w176) -> (w177:T18)
            n90 = call-poly <vilib>:"Delacor_lib_QMH_Enqueue Message (poly).vi"("Message Data"=w177, "Message"="mux10-1_chan8", "Message Queue in"=w180) -> ("error out"=w175:errorcluster)  [unwired: 7 in, 1 out]
          }
          event User Event {
            # "Another Module called the \"mux10-1_chan9\" API Method."
            n91 = event-data() -> ("Boolean"=w182:bool)  [unwired: 1 in]
            n92 = Bundle(cluster=T19 {"Boolean"=FALSE} ("mux10-1_chan9 Argument"), "Boolean"=w182) -> (w183:T19)
            n93 = call-poly <vilib>:"Delacor_lib_QMH_Enqueue Message (poly).vi"("Message Data"=w183, "Message"="mux10-1_chan9", "Message Queue in"=w186) -> ("error out"=w181:errorcluster)  [unwired: 7 in, 1 out]
          }
          event User Event {
            # "Another Module called the \"mux10-1_chan10\" API Method."
            n94 = event-data() -> ("Boolean"=w188:bool)  [unwired: 1 in]
            n95 = Bundle(cluster=T20 {"Boolean"=FALSE} ("mux10-1_chan10 Argument"), "Boolean"=w188) -> (w189:T20)
            n96 = call-poly <vilib>:"Delacor_lib_QMH_Enqueue Message (poly).vi"("Message Data"=w189, "Message"="mux10-1_chan10", "Message Queue in"=w192) -> ("error out"=w187:errorcluster)  [unwired: 7 in, 1 out]
          }
          event User Event {
            # "Another Module called the \"mux6-1_chan1_1\" API Method."
            n97 = event-data() -> ("Boolean"=w194:bool)  [unwired: 1 in]
            n98 = Bundle(cluster=T21 {"Boolean"=FALSE} ("mux6-1_chan1_1 Argument"), "Boolean"=w194) -> (w195:T21)
            n99 = call-poly <vilib>:"Delacor_lib_QMH_Enqueue Message (poly).vi"("Message Data"=w195, "Message"="mux6-1_chan1_1", "Message Queue in"=w198) -> ("error out"=w193:errorcluster)  [unwired: 7 in, 1 out]
          }
          event User Event {
            # "Another Module called the \"mux6-1_chan1_2\" API Method."
            n100 = event-data() -> ("Boolean"=w200:bool)  [unwired: 1 in]
            n101 = Bundle(cluster=T22 {"Boolean"=FALSE} ("mux6-1_chan1_2 Argument"), "Boolean"=w200) -> (w201:T22)
            n102 = call-poly <vilib>:"Delacor_lib_QMH_Enqueue Message (poly).vi"("Message Data"=w201, "Message"="mux6-1_chan1_2", "Message Queue in"=w204) -> ("error out"=w199:errorcluster)  [unwired: 7 in, 1 out]
          }
          event User Event {
            # "Another Module called the \"mux6-1_chan2_1\" API Method."
            n103 = event-data() -> ("Boolean"=w206:bool)  [unwired: 1 in]
            n104 = Bundle(cluster=T23 {"Boolean"=FALSE} ("mux6-1_chan2_1 Argument"), "Boolean"=w206) -> (w207:T23)
            n105 = call-poly <vilib>:"Delacor_lib_QMH_Enqueue Message (poly).vi"("Message Data"=w207, "Message"="mux6-1_chan2_1", "Message Queue in"=w210) -> ("error out"=w205:errorcluster)  [unwired: 7 in, 1 out]
          }
          event User Event {
            # "Another Module called the \"mux6-1_chan2_2\" API Method."
            n106 = event-data() -> ("Boolean"=w212:bool)  [unwired: 1 in]
            n107 = Bundle(cluster=T24 {"Boolean"=FALSE} ("mux6-1_chan2_2 Argument"), "Boolean"=w212) -> (w213:T24)
            n108 = call-poly <vilib>:"Delacor_lib_QMH_Enqueue Message (poly).vi"("Message Data"=w213, "Message"="mux6-1_chan2_2", "Message Queue in"=w216) -> ("error out"=w211:errorcluster)  [unwired: 7 in, 1 out]
          }
          event User Event {
            # "Another Module called the \"mux6-1_chan3_1\" API Method."
            n109 = event-data() -> ("Boolean"=w218:bool)  [unwired: 1 in]
            n110 = Bundle(cluster=T25 {"Boolean"=FALSE} ("mux6-1_chan3_1 Argument"), "Boolean"=w218) -> (w219:T25)
            n111 = call-poly <vilib>:"Delacor_lib_QMH_Enqueue Message (poly).vi"("Message Data"=w219, "Message"="mux6-1_chan3_1", "Message Queue in"=w222) -> ("error out"=w217:errorcluster)  [unwired: 7 in, 1 out]
          }
          event User Event {
            # "Another Module called the \"mux6-1_chan3_2\" API Method."
            n112 = event-data() -> ("Boolean"=w224:bool)  [unwired: 1 in]
            n113 = Bundle(cluster=T26 {"Boolean"=FALSE} ("mux6-1_chan3_2 Argument"), "Boolean"=w224) -> (w225:T26)
            n114 = call-poly <vilib>:"Delacor_lib_QMH_Enqueue Message (poly).vi"("Message Data"=w225, "Message"="mux6-1_chan3_2", "Message Queue in"=w228) -> ("error out"=w223:errorcluster)  [unwired: 7 in, 1 out]
          }
          event User Event {
            # "Another Module called the \"mux6-1_chan4_1\" API Method."
            n115 = event-data() -> ("Boolean"=w230:bool)  [unwired: 1 in]
            n116 = Bundle(cluster=T27 {"Boolean"=FALSE} ("mux6-1_chan4_1 Argument"), "Boolean"=w230) -> (w231:T27)
            n117 = call-poly <vilib>:"Delacor_lib_QMH_Enqueue Message (poly).vi"("Message Data"=w231, "Message"="mux6-1_chan4_1", "Message Queue in"=w234) -> ("error out"=w229:errorcluster)  [unwired: 7 in, 1 out]
          }
          event User Event {
            # "Another Module called the \"mux6-1_chan4_2\" API Method."
            n118 = event-data() -> ("Boolean"=w236:bool)  [unwired: 1 in]
            n119 = Bundle(cluster=T28 {"Boolean"=FALSE} ("mux6-1_chan4_2 Argument"), "Boolean"=w236) -> (w237:T28)
            n120 = call-poly <vilib>:"Delacor_lib_QMH_Enqueue Message (poly).vi"("Message Data"=w237, "Message"="mux6-1_chan4_2", "Message Queue in"=w240) -> ("error out"=w235:errorcluster)  [unwired: 7 in, 1 out]
          }
          event User Event {
            # "Another Module called the \"mux6-1_chan5_1\" API Method."
            n121 = event-data() -> ("Boolean"=w242:bool)  [unwired: 1 in]
            n122 = Bundle(cluster=T29 {"Boolean"=FALSE} ("mux6-1_chan5_1 Argument"), "Boolean"=w242) -> (w243:T29)
            n123 = call-poly <vilib>:"Delacor_lib_QMH_Enqueue Message (poly).vi"("Message Data"=w243, "Message"="mux6-1_chan5_1", "Message Queue in"=w246) -> ("error out"=w241:errorcluster)  [unwired: 7 in, 1 out]
          }
          event User Event {
            # "Another Module called the \"mux6-1_chan5_2\" API Method."
            n124 = event-data() -> ("Boolean"=w248:bool)  [unwired: 1 in]
            n125 = Bundle(cluster=T30 {"Boolean"=FALSE} ("mux6-1_chan5_2 Argument"), "Boolean"=w248) -> (w249:T30)
            n126 = call-poly <vilib>:"Delacor_lib_QMH_Enqueue Message (poly).vi"("Message Data"=w249, "Message"="mux6-1_chan5_2", "Message Queue in"=w252) -> ("error out"=w247:errorcluster)  [unwired: 7 in, 1 out]
          }
          event User Event {
            # "Another Module called the \"mux6-1_chan6_1\" API Method."
            n127 = event-data() -> ("Boolean"=w254:bool)  [unwired: 1 in]
            n128 = Bundle(cluster=T31 {"Boolean"=FALSE} ("mux6-1_chan6_1 Argument"), "Boolean"=w254) -> (w255:T31)
            n129 = call-poly <vilib>:"Delacor_lib_QMH_Enqueue Message (poly).vi"("Message Data"=w255, "Message"="mux6-1_chan6_1", "Message Queue in"=w258) -> ("error out"=w253:errorcluster)  [unwired: 7 in, 1 out]
          }
          event User Event {
            # "Another Module called the \"mux6-1_chan6_2\" API Method."
            n130 = event-data() -> ("Boolean"=w260:bool)  [unwired: 1 in]
            n131 = Bundle(cluster=T32 {"Boolean"=FALSE} ("mux6-1_chan6_2 Argument"), "Boolean"=w260) -> (w261:T32)
            n132 = call-poly <vilib>:"Delacor_lib_QMH_Enqueue Message (poly).vi"("Message Data"=w261, "Message"="mux6-1_chan6_2", "Message Queue in"=w264) -> ("error out"=w259:errorcluster)  [unwired: 7 in, 1 out]
          }
        }
        n133 = call-dynamic "Delacor_lib_QMH_Error Handler - Event Handling Loop.vi"("error in"=w32, "Message Queue in"=w26) -> ("dup error in"=w31:errorcluster)  [unwired: 8 in, 1 out]
      }
      n134 = while {
        tunnel: w19 -> [w267]
        shift-right: [w271] -> _
        shift-left: T2 {"Status"="", "Modbus Master ref"=refnum, "VISA resource name"=""} ("Data Cluster") -> [w272]
        tunnel: w23 -> [w275]
        tunnel: [w273] -> w25
        tunnel: w18 -> [w265]
        stop <- w270 stop-if-true
        # "Message Handling Loop"
        n135 = call-dynamic "Delacor_lib_QMH_Dequeue Message.vi"("error in"=w275, "Message Queue in"=w267) -> ("error out"=w274:errorcluster, "Message Data"=w268:variant, "Message"=w269:string, "Message Queue out"=w266:refnum<class "Delacor_lib_QMH_Message Queue.lvclass">)  [unwired: 6 in]
        n136 = case "DQMH_MESSAGE_CASES" shown="\"mux6-1_chan6_1\"" w269 {
          selector: w269 -> [_ _ _ _ _ _ _ _ _ _ _ _ _ _ _ _ _ _ _ _ _ _ _ _ _ _ _ _ _ _ _ _ _ _ _ _ _ w747]
          tunnel: w266 -> [_ _ _ _ _ _ _ _ _ _ _ _ _ _ _ _ _ _ _ _ _ _ _ _ _ _ _ _ _ _ _ _ _ _ _ w710 w733 _]
          tunnel: w274 -> [w297 w301 w320 w342 w353 w372 w395 w418 w430 w441 w452 w463 w474 w485 w496 w507 w518 w529 w540 w551 w562 w573 w584 w595 w607 w618 w629 w640 w652 w663 w674 w686 w693 w695 w700 w717 w739 w749]
          tunnel: [w279 w301 w319 w335 w347 w364 w387 w411 w424 w436 w447 w458 w469 w480 w491 w502 w513 w524 w535 w546 w557 w568 w579 w590 w601 w613 w624 w635 w646 w658 w669 w680 w692 w695 w699 w713 w736 w750] -> w276
          tunnel: w272 -> [w282 w300 w317 w333 w350 w363 w386 w414 w427 w437 w448 w459 w470 w481 w492 w503 w514 w525 w536 w548 w559 w569 w580 w591 w603 w614 w625 w636 w647 w659 w670 w681 w691 w694 w697 w712 w725 w748]
          tunnel: [w288 w300 w317 w337 w350 w363 w386 w414 w427 w437 w448 w459 w470 w481 w492 w503 w514 w525 w536 w548 w559 w569 w580 w591 w603 w614 w625 w636 w647 w659 w670 w681 w691 w694 w697 w712 w725 w748] -> w271
          tunnel: [_ _ _ _ _ _ _ _ _ _ _ _ _ _ _ _ _ _ _ _ _ _ _ _ _ _ _ _ _ _ _ _ _ _ _ _ w732 _] -> w270
          tunnel: w268 -> [_ _ w314 w341 w352 w371 w394 w417 w429 w439 w450 w461 w472 w483 w494 w505 w516 w527 w538 w550 w561 w571 w582 w593 w606 w616 w627 w638 w650 w661 w672 w684 _ _ _ w711 w731 _]
          tunnel: w265 -> [w289 _ _ _ _ _ _ _ _ _ _ _ _ _ _ _ _ _ _ _ _ _ _ _ _ _ _ _ _ _ _ _ _ _ _ w709 w726 _]
          frame "Initialize" {
            w277 = "Initial Message" ("Initial Message")
            # "Initialize - Any operation that needs to be done before the module can receive messages. Synchronize Caller Events.vi will inform Start Module.vi that the module has launched and is ready to receive messages. Module Did Init.vi will broadcast that the module initialized."
            n137 = call "Synchronize Caller Events.vi"("error in (no error)"=w297, "Singleton Module Admin in"=w289) -> ("error out"=w278:errorcluster, "Singleton Module Admin out"=w285:refnum<class "Delacor_lib_QMH_Module Admin.lvclass">)  [unwired: 8 in]
            n138 = property on="Pane" class="Pane"("Origin"=T33 {"Horizontal"=0, "Vertical"=0}) -> ()  [unwired: 2 in, 2 out]
            n139 = property class="Module Admin"(reference=w285) -> ("Accessors:External Launch"=w293:bool)  [unwired: 1 in, 2 out]
            n140 = Bundle By Name(cluster=w282, "VISA resource name"="VISA resource name") -> (w283:T2)
            n141 = call "Module Name--constant.vi"() -> ("Module Name"=w296:string)  [unwired: 11 in]
            n142 = Select(t=T34."Hidden" ("State"), s=w293, f=T34."Standard" ("State")) -> (s? t:f=w290:T34)
            n143 = property class="VI"("Front Panel.Title"=w296) -> (reference out=w295:refnum<vi>, error out=w299:errorcluster)  [unwired: 2 in]
            n144 = call "Module Name--constant.vi"() -> ("Module Name"=w286:string)  [unwired: 11 in]
            n145 = invoke class="VI" method="FP.Open"(reference=w295, error in=w299, "State"=w290) -> (reference out=w294:refnum<vi>, error out=w298:errorcluster)  [unwired: 2 in, 3 out]
            n146 = call "Module Did Init.vi"("error in (no error)"=w278, "Initialized?"=TRUE, "Origin"=w286) -> ("error out"=w280:errorcluster)  [unwired: 8 in]
            n147 = Bundle By Name(cluster=w283, "Status"=w277) -> (w288:T2)
            n148 = invoke class="VI" method="FP.Center"(reference=w294, error in=w298) -> ()  [unwired: 1 in, 3 out]
            n149 = Merge Errors(w280) -> (w279:errorcluster)
            "Status" <- w277
          }
          frame "---Module Specific---" {
            # "Separator -- The following cases handle messages specific to this Module."
          }
          frame "Do Something Else and Wait for Reply" {
            w309 = "X(%.2f)+Offset(%.2f)=%.2f"  # status message format string
            # "#DQMH_HowTo The 'Do Something' messages are instructional in nature and can be removed."
            # "Send back X with a random offset"
            # "Do Something Else and Wait for Reply - Replace this message with functionality for your own application. Note that this message must fire a notifier to let callers know it has finished execution, and it returns an error if the 'Value' is negative."
            n150 = Random Number (0-1)() -> (number: 0 to 1=w311:dbl)
            n151 = Variant To Data(error in=w320, type=T3 {"Do Something Else Msg"="", "X"=0.0, "Wait Notifier"=refnum, "wait for reply"=FALSE} ("Do Something Else and Wait for Reply Argument"), Variant=w314) -> (data=w315:T3, error out=w318:errorcluster)
            n152 = Unbundle By Name(w315) -> ("Wait Notifier"=w302:refnum<notifier>, "Do Something Else Msg"=w313:string, "X"=w310:dbl, "wait for reply"=w306:bool)
            n153 = Add(x=w311, y=w310) -> (x+y=w305:dbl)
            n154 = Less Than 0?(x=w305) -> (x < 0?=w308:bool)
            n155 = Format Into String(format string=w309, initial string=w313, w310, w311, w305) -> (resulting string=w307:string)  [unwired: 1 in, 1 out]
            n156 = case shown="True" w308 {
              tunnel: [_ w327] -> w303
              frame False {
              }
              frame True {
                n157 = xnode "Error Ring"() -> ("error out"=w327:errorcluster)
              }
            }
            n158 = Bundle By Name(cluster=T35 {"Value"=0.0, "error"={"status"=FALSE, "code"=0, "source"=""}} ("notification"), "error"=w303, "Value"=w305) -> (w304:T35)
            n159 = local write "Status"(w307) -> ()
            n160 = call "Status Updated.vi"("Status"=w307) -> ()  [unwired: 10 in, 1 out]
            n161 = case shown="True" w306 {
              tunnel: w304 -> [_ w323]
              tunnel: w302 -> [_ w322]
              frame False {
              }
              frame True {
                # "Simulate an operation that requires a wait."
                n162 = flat-sequence {
                  tunnel: w323 -> [w326]
                  tunnel: w322 -> [w325]
                  tunnel: w321 -> [_]
                  frame #0 {
                    n163 = Send Notification(notification=w326, notifier=w325) -> ()  [unwired: 1 in, 2 out]
                  }
                }
                n164 = Wait (ms)(milliseconds to wait=u32 1000) -> (millisecond timer value=w321:u32)
              }
            }
            n165 = Merge Errors(w318, w303) -> (w319:errorcluster)
          }
          frame "inst.Open" {
            # "send COMport name to Module and Open Modbus Insstance"
            n166 = Variant To Data(error in=w342, type=T36 {"VISA resource name"=""} ("Open COM Argument"), Variant=w341) -> (error out=w334:errorcluster)  [unwired: 1 out]
            n167 = Unbundle By Name(w333) -> ("VISA resource name"=w339:refnum<visa-resource-name>)
            n168 = disable-structure shown="NO_HARDWARE==TRUE" {
              disable-tunnel: w339 -> [w346 _]
              disable-tunnel: [w345 _] -> w338
              disable-tunnel: [w344 _] -> w336
              frame condition #0 {
                n169 = call "inst.Open.vi"("unit ID in"=u8 21, "VISA resource name"=w346) -> ("error out"=w344:errorcluster, "Modbus Master out"=w345:refnum<class "Modbus Master.lvclass">)  [unwired: 8 in]
              }
              frame condition #1 (active) {
              }
            }
            n170 = Bundle By Name(cluster=w333, "Modbus Master ref"=w338) -> (w337:T2)
            n171 = Merge Errors(w334, w336) -> (w335:errorcluster)
          }
          frame "inst.Close" {
            # "Shut down all Relays and Close COM port"
            n172 = Variant To Data(error in=w353, type=T37 {"Boolean"=FALSE} ("Close COM Argument"), Variant=w352) -> (error out=w349:errorcluster)  [unwired: 1 out]
            n173 = disable-structure shown="NO_HARDWARE==TRUE" {
              disable-tunnel: w350 -> [w357 _]
              disable-tunnel: [w354 _] -> w348
              frame condition #0 {
                n174 = Unbundle By Name(w357) -> ("Modbus Master ref"=w359:refnum<class "Modbus Master.lvclass">)
                n175 = call "FGV_HoldingRegs.vi"("FGV_enum"=FGV_enum."All OFF", "Modbus master in"=w359) -> ("error out"=w356:errorcluster, "Modbus master out"=w355:refnum<class "Modbus Master.lvclass">)  [unwired: 7 in, 1 out]
                n176 = call "inst.Close (SubVI).vi"("error in (no error)"=w356, "Modbus Master in"=w355) -> ("error out"=w354:errorcluster)  [unwired: 9 in]
              }
              frame condition #1 (active) {
              }
            }
            n177 = Merge Errors(w349, w348) -> (w347:errorcluster)
          }
          frame "inst.Counter" {
            # "Read Internal Counter to check state of MCU"
            n178 = disable-structure shown="Default" {
              disable-tunnel: w363 -> [w377 _]
              disable-tunnel: [w375 w380] -> w360
              disable-tunnel: [w374 _] -> w361
              frame condition #0 {
                n179 = Unbundle By Name(w377) -> ("Modbus Master ref"=w376:refnum<class "Modbus Master.lvclass">)
                n180 = call "inst.counter.vi"("unit ID(1)"=u8 21, "Modbus master in"=w376) -> ("error out"=w374:errorcluster, "counter"=w375:u16)  [unwired: 7 in, 1 out]
              }
              frame condition #1 (active) {
                n181 = feedback #1(u16 0) -> (w378:u16)
                n182 = Increment(x=w378) -> (x+1=w380:u16)
                n183 = feedback-in #1(w380) -> ()
              }
            }
            n184 = Variant To Data(error in=w372, type=T6 {"Wait Notifier"=refnum, "wait for reply"=FALSE} ("Read Counter Argument"), Variant=w371) -> (data=w369:T6, error out=w362:errorcluster)
            n185 = Unbundle By Name(w369) -> ("Wait Notifier"=w368:refnum<notifier>, "wait for reply"=w367:bool)
            n186 = Bundle By Name(cluster=T39 {"counter"=0, "inst.Counter_error"={"status"=FALSE, "code"=0, "source"=""}} ("Read Counter (Reply Payload)"), "counter"=w360) -> (w366:T39)
            n187 = case shown="True" w367 {
              tunnel: w368 -> [_ w382]
              tunnel: w366 -> [_ w381]
              frame False {
              }
              frame True {
                n188 = Send Notification(notification=w381, notifier=w382) -> ()  [unwired: 1 in, 2 out]
              }
            }
            n189 = Merge Errors(w362, w361) -> (w364:errorcluster)
          }
          frame "inst.Optos" {
            # "Read 60 optos DIs"
            n190 = disable-structure shown="NO_HARDWARE==TRUE" {
              disable-tunnel: w386 -> [w399 _]
              disable-tunnel: [w397 _] -> w384
              disable-tunnel: [w396 w400] -> w383
              frame condition #0 {
                n191 = Unbundle By Name(w399) -> ("Modbus Master ref"=w398:refnum<class "Modbus Master.lvclass">)
                n192 = call "inst.Optos.vi"("Modbus master in"=w398) -> ("error out"=w397:errorcluster, "optos"=w396:bool[])  [unwired: 8 in, 1 out]
              }
              frame condition #1 (active) {
                w403 = TRUE
                n193 = Initialize Array(FALSE, 60 ("dimension size")) -> (w401:bool[])
                n194 = Replace Array Subset(array=w401, new element #1=w403, index #1=6 ("index"), new element #2=w403, index #2=13 ("index"), new element #3=w403, index #3=27 ("index"), new element #4=w403, index #4=32 ("index")) -> (w400:bool[])
              }
            }
            n195 = Variant To Data(error in=w395, type=T7 {"Wait Notifier"=refnum, "wait for reply"=FALSE} ("Read Optos Argument"), Variant=w394) -> (data=w392:T7, error out=w385:errorcluster)
            n196 = Unbundle By Name(w392) -> ("Wait Notifier"=w391:refnum<notifier>, "wait for reply"=w390:bool)
            n197 = Merge Errors(w385, w384) -> (w387:errorcluster)
            n198 = Bundle By Name(cluster=T40 {"Optos"=[], "inst.Optos_error"={"status"=FALSE, "code"=0, "source"=""}} ("Read Optos (Reply Payload)"), "Optos"=w383) -> (w389:T40)
            n199 = case shown="True" w390 {
              tunnel: w391 -> [_ w410]
              tunnel: w389 -> [_ w409]
              frame False {
              }
              frame True {
                n200 = Send Notification(notification=w409, notifier=w410) -> ()  [unwired: 1 in, 2 out]
              }
            }
          }
          frame "DMM I 0.5_10" {
            # "DMM config Current fuse 0.5 or 10A"
            n201 = Variant To Data(error in=w418, type=T10 {"mux2-1(DMM I) encode"=enum."DMM I (0.5)"} ("DMM I 0.5_10 Argument"), Variant=w417) -> (data=w415:T10, error out=w413:errorcluster)
            n202 = disable-structure shown="Default" {
              disable-tunnel: w415 -> [w423 _]
              disable-tunnel: w414 -> [w422 _]
              disable-tunnel: [w420 _] -> w412
              frame condition #0 {
                n203 = Unbundle By Name(w423) -> ("mux2-1(DMM I) encode"=w419:enum16{"DMM I (0.5)", "DMM I (12)"})
                n204 = Unbundle By Name(w422) -> ("Modbus Master ref"=w421:refnum<class "Modbus Master.lvclass">)
                n205 = call "inst.DMM (Current INPUT).vi"("mux2-1(DMM I) encode"=w419, "Modbus Master in"=w421) -> ("error out"=w420:errorcluster)  [unwired: 8 in, 1 out]
              }
              frame condition #1 (active) {
              }
            }
            n206 = Merge Errors(w413, w412) -> (w411:errorcluster)
          }
          frame "mux10-1_chan0" {
            # "Connect DRV output to LED loads"
            n207 = Variant To Data(error in=w430, type=T8 {"mux10_1(x6)_encode"=enum."mux10_1_channel0"} ("inst.mux10_1 Argument"), Variant=w429) -> (error out=w425:errorcluster)  [unwired: 1 out]
            n208 = disable-structure shown="Default" {
              disable-tunnel: w427 -> [w434 _]
              disable-tunnel: [w432 _] -> w426
              frame condition #0 {
                n209 = Unbundle By Name(w434) -> ("Modbus Master ref"=w433:refnum<class "Modbus Master.lvclass">)
                n210 = call "inst.mux10.1(x6).vi"("mux10_1(x6)_encode"=T41."mux10_1_channel0", "Modbus Master in"=w433) -> ("error out"=w432:errorcluster)  [unwired: 8 in, 1 out]
              }
              frame condition #1 (active) {
              }
            }
            n211 = Merge Errors(w425, w426) -> (w424:errorcluster)
          }
          frame "mux10-1_chan1" {
            n212 = Variant To Data(error in=w441, type=T11 {"Boolean"=FALSE} ("mux10-1_chan1 Argument"), Variant=w439) -> (error out=w440:errorcluster)  [unwired: 1 out]
            n213 = disable-structure shown="Default" {
              disable-tunnel: w437 -> [w445]
              disable-tunnel: [w442] -> w435
              frame Enabled {
                n214 = Unbundle By Name(w445) -> ("Modbus Master ref"=w444:refnum<class "Modbus Master.lvclass">)
                n215 = call "inst.mux10.1(x6).vi"("mux10_1(x6)_encode"=T41."mux10_1_channel1", "Modbus Master in"=w444) -> ("error out"=w442:errorcluster)  [unwired: 8 in, 1 out]
              }
            }
            n216 = Merge Errors(w440, w435) -> (w436:errorcluster)
          }
          frame "mux10-1_chan2" {
            n217 = Variant To Data(error in=w452, type=T12 {"Boolean"=FALSE} ("mux10-1_chan2 Argument"), Variant=w450) -> (error out=w451:errorcluster)  [unwired: 1 out]
            n218 = disable-structure shown="Default" {
              disable-tunnel: w448 -> [w456]
              disable-tunnel: [w453] -> w446
              frame Enabled {
                n219 = Unbundle By Name(w456) -> ("Modbus Master ref"=w455:refnum<class "Modbus Master.lvclass">)
                n220 = call "inst.mux10.1(x6).vi"("mux10_1(x6)_encode"=T41."mux10_1_channel2", "Modbus Master in"=w455) -> ("error out"=w453:errorcluster)  [unwired: 8 in, 1 out]
              }
            }
            n221 = Merge Errors(w451, w446) -> (w447:errorcluster)
          }
          frame "mux10-1_chan3" {
            n222 = Variant To Data(error in=w463, type=T13 {"Boolean"=FALSE} ("mux10-1_chan3 Argument"), Variant=w461) -> (error out=w462:errorcluster)  [unwired: 1 out]
            n223 = disable-structure shown="Default" {
              disable-tunnel: w459 -> [w467]
              disable-tunnel: [w464] -> w457
              frame Enabled {
                n224 = Unbundle By Name(w467) -> ("Modbus Master ref"=w466:refnum<class "Modbus Master.lvclass">)
                n225 = call "inst.mux10.1(x6).vi"("mux10_1(x6)_encode"=T41."mux10_1_channel3", "Modbus Master in"=w466) -> ("error out"=w464:errorcluster)  [unwired: 8 in, 1 out]
              }
            }
            n226 = Merge Errors(w462, w457) -> (w458:errorcluster)
          }
          frame "mux10-1_chan4" {
            n227 = Variant To Data(error in=w474, type=T14 {"Boolean"=FALSE} ("mux10-1_chan4 Argument"), Variant=w472) -> (error out=w473:errorcluster)  [unwired: 1 out]
            n228 = disable-structure shown="Default" {
              disable-tunnel: w470 -> [w478]
              disable-tunnel: [w475] -> w468
              frame Enabled {
                n229 = Unbundle By Name(w478) -> ("Modbus Master ref"=w477:refnum<class "Modbus Master.lvclass">)
                n230 = call "inst.mux10.1(x6).vi"("mux10_1(x6)_encode"=T41."mux10_1_channel4", "Modbus Master in"=w477) -> ("error out"=w475:errorcluster)  [unwired: 8 in, 1 out]
              }
            }
            n231 = Merge Errors(w473, w468) -> (w469:errorcluster)
          }
          frame "mux10-1_chan5" {
            n232 = Variant To Data(error in=w485, type=T15 {"Boolean"=FALSE} ("mux10-1_chan5 Argument"), Variant=w483) -> (error out=w484:errorcluster)  [unwired: 1 out]
            n233 = disable-structure shown="Default" {
              disable-tunnel: w481 -> [w489]
              disable-tunnel: [w487] -> w479
              frame Enabled {
                n234 = Unbundle By Name(w489) -> ("Modbus Master ref"=w488:refnum<class "Modbus Master.lvclass">)
                n235 = call "inst.mux10.1(x6).vi"("mux10_1(x6)_encode"=T41."mux10_1_channel5", "Modbus Master in"=w488) -> ("error out"=w487:errorcluster)  [unwired: 8 in, 1 out]
              }
            }
            n236 = Merge Errors(w484, w479) -> (w480:errorcluster)
          }
          frame "mux10-1_chan6" {
            n237 = Variant To Data(error in=w496, type=T16 {"Boolean"=FALSE} ("mux10-1_chan6 Argument"), Variant=w494) -> (error out=w495:errorcluster)  [unwired: 1 out]
            n238 = disable-structure shown="Default" {
              disable-tunnel: w492 -> [w500]
              disable-tunnel: [w497] -> w490
              frame Enabled {
                n239 = Unbundle By Name(w500) -> ("Modbus Master ref"=w499:refnum<class "Modbus Master.lvclass">)
                n240 = call "inst.mux10.1(x6).vi"("mux10_1(x6)_encode"=T41."mux10_1_channel6", "Modbus Master in"=w499) -> ("error out"=w497:errorcluster)  [unwired: 8 in, 1 out]
              }
            }
            n241 = Merge Errors(w495, w490) -> (w491:errorcluster)
          }
          frame "mux10-1_chan7" {
            n242 = Variant To Data(error in=w507, type=T17 {"Boolean"=FALSE} ("mux10-1_chan7 Argument"), Variant=w505) -> (error out=w506:errorcluster)  [unwired: 1 out]
            n243 = disable-structure shown="Default" {
              disable-tunnel: w503 -> [w511]
              disable-tunnel: [w509] -> w501
              frame Enabled {
                n244 = Unbundle By Name(w511) -> ("Modbus Master ref"=w510:refnum<class "Modbus Master.lvclass">)
                n245 = call "inst.mux10.1(x6).vi"("mux10_1(x6)_encode"=T41."mux10_1_channel7", "Modbus Master in"=w510) -> ("error out"=w509:errorcluster)  [unwired: 8 in, 1 out]
              }
            }
            n246 = Merge Errors(w506, w501) -> (w502:errorcluster)
          }
          frame "mux10-1_chan8" {
            n247 = Variant To Data(error in=w518, type=T18 {"Boolean"=FALSE} ("mux10-1_chan8 Argument"), Variant=w516) -> (error out=w517:errorcluster)  [unwired: 1 out]
            n248 = disable-structure shown="Default" {
              disable-tunnel: w514 -> [w522]
              disable-tunnel: [w520] -> w512
              frame Enabled {
                n249 = Unbundle By Name(w522) -> ("Modbus Master ref"=w521:refnum<class "Modbus Master.lvclass">)
                n250 = call "inst.mux10.1(x6).vi"("mux10_1(x6)_encode"=T41."mux10_1_channel8", "Modbus Master in"=w521) -> ("error out"=w520:errorcluster)  [unwired: 8 in, 1 out]
              }
            }
            n251 = Merge Errors(w517, w512) -> (w513:errorcluster)
          }
          frame "mux10-1_chan9" {
            n252 = Variant To Data(error in=w529, type=T19 {"Boolean"=FALSE} ("mux10-1_chan9 Argument"), Variant=w527) -> (error out=w528:errorcluster)  [unwired: 1 out]
            n253 = disable-structure shown="Default" {
              disable-tunnel: w525 -> [w533]
              disable-tunnel: [w531] -> w523
              frame Enabled {
                n254 = Unbundle By Name(w533) -> ("Modbus Master ref"=w532:refnum<class "Modbus Master.lvclass">)
                n255 = call "inst.mux10.1(x6).vi"("mux10_1(x6)_encode"=T41."mux10_1_channel9", "Modbus Master in"=w532) -> ("error out"=w531:errorcluster)  [unwired: 8 in, 1 out]
              }
            }
            n256 = Merge Errors(w528, w523) -> (w524:errorcluster)
          }
          frame "mux10-1_chan10" {
            n257 = Variant To Data(error in=w540, type=T20 {"Boolean"=FALSE} ("mux10-1_chan10 Argument"), Variant=w538) -> (error out=w539:errorcluster)  [unwired: 1 out]
            n258 = disable-structure shown="NO_HARDWARE==TRUE" {
              disable-tunnel: w536 -> [w544 _]
              disable-tunnel: [w542 _] -> w534
              frame condition #0 {
                n259 = Unbundle By Name(w544) -> ("Modbus Master ref"=w543:refnum<class "Modbus Master.lvclass">)
                n260 = call "inst.mux10.1(x6).vi"("mux10_1(x6)_encode"=T41."mux10_1_channel10", "Modbus Master in"=w543) -> ("error out"=w542:errorcluster)  [unwired: 8 in, 1 out]
              }
              frame condition #1 (active) {
              }
            }
            n261 = Merge Errors(w539, w534) -> (w535:errorcluster)
          }
          frame "mux6-1_chan0" {
            # "connect Led DRV to DMM inputs"
            n262 = Variant To Data(error in=w551, type=T9 {"mux6_1(3wires)_encode"=enum."mux6-1_channel0"} ("inst.mux6_1(3wires) Argument"), Variant=w550) -> (error out=w547:errorcluster)  [unwired: 1 out]
            n263 = disable-structure shown="Default" {
              disable-tunnel: w548 -> [w555 _]
              disable-tunnel: [w553 _] -> w545
              frame condition #0 {
                n264 = Unbundle By Name(w555) -> ("Modbus Master ref"=w554:refnum<class "Modbus Master.lvclass">)
                n265 = call "inst.mux6.1(3wires).vi"("mux6_1(3wires)_encode"=T42."mux6-1_channel0", "Modbus Master in"=w554) -> ("error out"=w553:errorcluster)  [unwired: 8 in, 1 out]
              }
              frame condition #1 (active) {
              }
            }
            n266 = Merge Errors(w547, w545) -> (w546:errorcluster)
          }
          frame "mux6-1_chan1_1" {
            n267 = Variant To Data(error in=w562, type=T21 {"Boolean"=FALSE} ("mux6-1_chan1_1 Argument"), Variant=w561) -> (error out=w558:errorcluster)  [unwired: 1 out]
            n268 = disable-structure shown="Default" {
              disable-tunnel: w559 -> [w566]
              disable-tunnel: [w563] -> w556
              frame Enabled {
                n269 = Unbundle By Name(w566) -> ("Modbus Master ref"=w565:refnum<class "Modbus Master.lvclass">)
                n270 = call "inst.mux6.1(3wires).vi"("mux6_1(3wires)_encode"=T42."mux6-1_channel1_2", "Modbus Master in"=w565) -> ("error out"=w563:errorcluster)  [unwired: 8 in, 1 out]
              }
            }
            n271 = Merge Errors(w558, w556) -> (w557:errorcluster)
          }
          frame "mux6-1_chan1_2" {
            n272 = Variant To Data(error in=w573, type=T22 {"Boolean"=FALSE} ("mux6-1_chan1_2 Argument"), Variant=w571) -> (error out=w572:errorcluster)  [unwired: 1 out]
            n273 = disable-structure shown="Default" {
              disable-tunnel: w569 -> [w577]
              disable-tunnel: [w574] -> w567
              frame Enabled {
                n274 = Unbundle By Name(w577) -> ("Modbus Master ref"=w576:refnum<class "Modbus Master.lvclass">)
                n275 = call "inst.mux6.1(3wires).vi"("mux6_1(3wires)_encode"=T42."mux6_1_channel1_3", "Modbus Master in"=w576) -> ("error out"=w574:errorcluster)  [unwired: 8 in, 1 out]
              }
            }
            n276 = Merge Errors(w572, w567) -> (w568:errorcluster)
          }
          frame "mux6-1_chan2_1" {
            n277 = Variant To Data(error in=w584, type=T23 {"Boolean"=FALSE} ("mux6-1_chan2_1 Argument"), Variant=w582) -> (error out=w583:errorcluster)  [unwired: 1 out]
            n278 = disable-structure shown="Default" {
              disable-tunnel: w580 -> [w588]
              disable-tunnel: [w585] -> w578
              frame Enabled {
                n279 = Unbundle By Name(w588) -> ("Modbus Master ref"=w587:refnum<class "Modbus Master.lvclass">)
                n280 = call "inst.mux6.1(3wires).vi"("mux6_1(3wires)_encode"=T42."mux6_1_channel2_2", "Modbus Master in"=w587) -> ("error out"=w585:errorcluster)  [unwired: 8 in, 1 out]
              }
            }
            n281 = Merge Errors(w583, w578) -> (w579:errorcluster)
          }
          frame "mux6-1_chan2_2" {
            n282 = Variant To Data(error in=w595, type=T24 {"Boolean"=FALSE} ("mux6-1_chan2_2 Argument"), Variant=w593) -> (error out=w594:errorcluster)  [unwired: 1 out]
            n283 = disable-structure shown="Default" {
              disable-tunnel: w591 -> [w599]
              disable-tunnel: [w596] -> w589
              frame Enabled {
                n284 = Unbundle By Name(w599) -> ("Modbus Master ref"=w598:refnum<class "Modbus Master.lvclass">)
                n285 = call "inst.mux6.1(3wires).vi"("mux6_1(3wires)_encode"=T42."mux6_1_channel2_3", "Modbus Master in"=w598) -> ("error out"=w596:errorcluster)  [unwired: 8 in, 1 out]
              }
            }
            n286 = Merge Errors(w594, w589) -> (w590:errorcluster)
          }
          frame "mux6-1_chan3_1" {
            n287 = Variant To Data(error in=w607, type=T25 {"Boolean"=FALSE} ("mux6-1_chan3_1 Argument"), Variant=w606) -> (data=w604:T25, error out=w602:errorcluster)
            n288 = disable-structure shown="Default" {
              disable-tunnel: w603 -> [w611]
              disable-tunnel: [w608] -> w600
              frame Enabled {
                n289 = Unbundle By Name(w611) -> ("Modbus Master ref"=w610:refnum<class "Modbus Master.lvclass">)
                n290 = call "inst.mux6.1(3wires).vi"("mux6_1(3wires)_encode"=T42."mux6_1_channel3_2", "Modbus Master in"=w610) -> ("error out"=w608:errorcluster)  [unwired: 8 in, 1 out]
              }
            }
            n291 = Unbundle By Name(w604) -> ()  [unwired: 1 out]
            n292 = Merge Errors(w602, w600) -> (w601:errorcluster)
          }
          frame "mux6-1_chan3_2" {
            n293 = Variant To Data(error in=w618, type=T26 {"Boolean"=FALSE} ("mux6-1_chan3_2 Argument"), Variant=w616) -> (error out=w617:errorcluster)  [unwired: 1 out]
            n294 = disable-structure shown="Default" {
              disable-tunnel: w614 -> [w622]
              disable-tunnel: [w619] -> w612
              frame Enabled {
                n295 = Unbundle By Name(w622) -> ("Modbus Master ref"=w621:refnum<class "Modbus Master.lvclass">)
                n296 = call "inst.mux6.1(3wires).vi"("mux6_1(3wires)_encode"=T42."mux6_1_channel3_3", "Modbus Master in"=w621) -> ("error out"=w619:errorcluster)  [unwired: 8 in, 1 out]
              }
            }
            n297 = Merge Errors(w617, w612) -> (w613:errorcluster)
          }
          frame "mux6-1_chan4_1" {
            n298 = Variant To Data(error in=w629, type=T27 {"Boolean"=FALSE} ("mux6-1_chan4_1 Argument"), Variant=w627) -> (error out=w628:errorcluster)  [unwired: 1 out]
            n299 = disable-structure shown="Default" {
              disable-tunnel: w625 -> [w633]
              disable-tunnel: [w630] -> w623
              frame Enabled {
                n300 = Unbundle By Name(w633) -> ("Modbus Master ref"=w632:refnum<class "Modbus Master.lvclass">)
                n301 = call "inst.mux6.1(3wires).vi"("mux6_1(3wires)_encode"=T42."mux6_1_channel4_2", "Modbus Master in"=w632) -> ("error out"=w630:errorcluster)  [unwired: 8 in, 1 out]
              }
            }
            n302 = Merge Errors(w628, w623) -> (w624:errorcluster)
          }
          frame "mux6-1_chan4_2" {
            n303 = Variant To Data(error in=w640, type=T28 {"Boolean"=FALSE} ("mux6-1_chan4_2 Argument"), Variant=w638) -> (error out=w639:errorcluster)  [unwired: 1 out]
            n304 = disable-structure shown="Default" {
              disable-tunnel: w636 -> [w644]
              disable-tunnel: [w641] -> w634
              frame Enabled {
                n305 = Unbundle By Name(w644) -> ("Modbus Master ref"=w643:refnum<class "Modbus Master.lvclass">)
                n306 = call "inst.mux6.1(3wires).vi"("mux6_1(3wires)_encode"=T42."mux6_1_channel4_3", "Modbus Master in"=w643) -> ("error out"=w641:errorcluster)  [unwired: 8 in, 1 out]
              }
            }
            n307 = Merge Errors(w639, w634) -> (w635:errorcluster)
          }
          frame "mux6-1_chan5_1" {
            n308 = Variant To Data(error in=w652, type=T29 {"Boolean"=FALSE} ("mux6-1_chan5_1 Argument"), Variant=w650) -> (data=w648:T29, error out=w651:errorcluster)
            n309 = disable-structure shown="Default" {
              disable-tunnel: w647 -> [w656]
              disable-tunnel: [w653] -> w645
              frame Enabled {
                n310 = Unbundle By Name(w656) -> ("Modbus Master ref"=w655:refnum<class "Modbus Master.lvclass">)
                n311 = call "inst.mux6.1(3wires).vi"("mux6_1(3wires)_encode"=T42."mux6_1_channel5_2", "Modbus Master in"=w655) -> ("error out"=w653:errorcluster)  [unwired: 8 in, 1 out]
              }
            }
            n312 = Unbundle By Name(w648) -> ()  [unwired: 1 out]
            n313 = Merge Errors(w651, w645) -> (w646:errorcluster)
          }
          frame "mux6-1_chan5_2" {
            n314 = Variant To Data(error in=w663, type=T30 {"Boolean"=FALSE} ("mux6-1_chan5_2 Argument"), Variant=w661) -> (error out=w662:errorcluster)  [unwired: 1 out]
            n315 = disable-structure shown="Default" {
              disable-tunnel: w659 -> [w667]
              disable-tunnel: [w664] -> w657
              frame Enabled {
                n316 = Unbundle By Name(w667) -> ("Modbus Master ref"=w666:refnum<class "Modbus Master.lvclass">)
                n317 = call "inst.mux6.1(3wires).vi"("mux6_1(3wires)_encode"=T42."mux6_1_channel5_3", "Modbus Master in"=w666) -> ("error out"=w664:errorcluster)  [unwired: 8 in, 1 out]
              }
            }
            n318 = Merge Errors(w662, w657) -> (w658:errorcluster)
          }
          frame "mux6-1_chan6_1" {
            n319 = Variant To Data(error in=w674, type=T31 {"Boolean"=FALSE} ("mux6-1_chan6_1 Argument"), Variant=w672) -> (error out=w673:errorcluster)  [unwired: 1 out]
            n320 = disable-structure shown="Default" {
              disable-tunnel: w670 -> [w678]
              disable-tunnel: [w675] -> w668
              frame Enabled {
                n321 = Unbundle By Name(w678) -> ("Modbus Master ref"=w677:refnum<class "Modbus Master.lvclass">)
                n322 = call "inst.mux6.1(3wires).vi"("mux6_1(3wires)_encode"=T42."mux6_1_channel6_2", "Modbus Master in"=w677) -> ("error out"=w675:errorcluster)  [unwired: 8 in, 1 out]
              }
            }
            n323 = Merge Errors(w673, w668) -> (w669:errorcluster)
          }
          frame "mux6-1_chan6_2" {
            n324 = Variant To Data(error in=w686, type=T32 {"Boolean"=FALSE} ("mux6-1_chan6_2 Argument"), Variant=w684) -> (data=w682:T32, error out=w685:errorcluster)
            n325 = disable-structure shown="Default" {
              disable-tunnel: w681 -> [w690]
              disable-tunnel: [w687] -> w679
              frame Enabled {
                n326 = Unbundle By Name(w690) -> ("Modbus Master ref"=w689:refnum<class "Modbus Master.lvclass">)
                n327 = call "inst.mux6.1(3wires).vi"("mux6_1(3wires)_encode"=T42."mux6_1_channel6_3", "Modbus Master in"=w689) -> ("error out"=w687:errorcluster)  [unwired: 8 in, 1 out]
              }
            }
            n328 = Unbundle By Name(w682) -> ()  [unwired: 1 out]
            n329 = Merge Errors(w685, w679) -> (w680:errorcluster)
          }
          frame "---Copy This Frame---" {
            # "Duplicate this frame when creating new messages.  Change this comment in the duplicated frame to describe this message."
            n330 = Merge Errors(w693) -> (w692:errorcluster)
          }
          frame "---Exit and Error Handling---" {
            # "Separator - The following cases handle errors and exit messages."
          }
          frame "Simulate MHL Error" {
            # "#DQMH_HowTo The 'Simulate MHL Error' button  illustrates how the MHL handles errors. This event is instructional in nature and can be removed."
            # "Simulate an error occurring at the MHL"
            n331 = call "Module Name--constant.vi"() -> ("Module Name"=w696:string)  [unwired: 11 in]
            n332 = xnode "Error Ring"("parameter 0"=w696) -> ("error out"=w698:errorcluster)
            n333 = Merge Errors(w700, w698) -> (w699:errorcluster)
          }
          frame "Error" {
            # "#CodeRecommended - If you ever change the name of this \"Error\" message, you'll need to update the name in the Check Loop Error.vi as well."
            # "#CodeRecommended - If the module is running in standalone mode (External Launch = FALSE), this code will pop up an error dialog and call the 'Exit' message if an error occurs. Add more fine-grained error handling here."
            # "Error - Check the error message data and respond accordingly. This message is sent by the \"Error Handler\" VIs at the end of each loop in this application."
            n334 = property class="Module Admin"(reference=w709) -> ("Accessors:External Launch"=w708:bool)  [unwired: 1 in, 2 out]
            n335 = Variant To Data(error in=w717, type=errorcluster {"status"=FALSE, "code"=0, "source"=""} ("error constant"), Variant=w711) -> (data=w718:errorcluster, error out=w715:errorcluster)
            n336 = call "Error Reported.vi"("Error"=w718) -> ()  [unwired: 10 in, 1 out]
            n337 = case shown="False" w708 {
              tunnel: [w723 _] -> w714
              tunnel: w710 -> [w721 _]
              tunnel: w718 -> [w722 _]
              frame False {
                # "If the module is running standalone, then pop up an error dialog and call the \"Exit\" message."
                n338 = call <vilib>:"Simple Error Handler.vi"("error in (no error)"=w722) -> ()  [unwired: 4 in, 5 out]
                n339 = call-poly <vilib>:"Delacor_lib_QMH_Enqueue Message (poly).vi"("Priority Message? (F)"=TRUE, "Message"="Exit", "Message Queue in"=w721) -> ("error out"=w723:errorcluster)  [unwired: 7 in, 1 out]
              }
              frame True {
                # "If the module was launched externally, calling the Error Reported broadcast VI is the only action performed by the \"Error\" message. The module's caller can then process the error appropriately."
              }
            }
            n340 = Merge Errors(w715, w714) -> (w713:errorcluster)
            n341 = local write "error out"(w713) -> ()
          }
          frame "Exit" {
            w730 = 91  # 91: not all Exit messages will have an argument
            w732 = TRUE  # Stop the VI
            # "Release the message queue reference"
            # "Exit - Exit the application."
            n342 = Variant To Data(error in=w739, type=T5 {"Origin"="", "Exit via Stop Module Req?"=FALSE, "Wait for Module to stop?"=FALSE} ("Stop Argument"), Variant=w731) -> (data=w728:T5, error out=w735:errorcluster)
            n343 = call <vilib>:"Clear Errors.vi"("error in (no error)"=w735, "specific error code to clear (0: all)"=w730) -> ("error out"=w738:errorcluster)  [unwired: 4 in, 1 out]
            n344 = disable-structure shown="Default" {
              disable-tunnel: w725 -> [w741 _]
              disable-tunnel: [w740 _] -> w724
              frame condition #0 {
                n345 = Unbundle By Name(w741) -> ("Modbus Master ref"=w745:refnum<class "Modbus Master.lvclass">)
                n346 = call "FGV_HoldingRegs.vi"("FGV_enum"=FGV_enum."All OFF", "Modbus master in"=w745) -> ("error out"=w744:errorcluster, "Modbus master out"=w743:refnum<class "Modbus Master.lvclass">)  [unwired: 7 in, 1 out]
                n347 = call "inst.Close (SubVI).vi"("error in (no error)"=w744, "Modbus Master in"=w743) -> ("error out"=w740:errorcluster)  [unwired: 9 in]
              }
              frame condition #1 (active) {
              }
            }
            n348 = control-ref of="This VI"() -> (w727:refnum<vi>)
            n349 = call-dynamic "Delacor_lib_QMH_Release Message Queue.vi"("error in"=w738, "Message Queue"=w733) -> ("error out"=w737:errorcluster)  [unwired: 9 in]
            n350 = call "Handle Exit.vi"("Stop Argument"=w728, "Admin in"=w726, "VI reference"=w727) -> ("error out"=w734:errorcluster)  [unwired: 7 in, 1 out]
            n351 = Merge Errors(w737, w734, w724) -> (w736:errorcluster)
          }
          frame Default {
            # "'Default' case only runs if there is a message that isn't defined in any of the other cases.  Output a programming error."
            n352 = call "Module Name--constant.vi"() -> ("Module Name"=w746:string)  [unwired: 11 in]
            n353 = xnode "Error Ring"("parameter 0"=w747, "parameter 1"=w746) -> ("error out"=w751:errorcluster)
            n354 = Merge Errors(w749, w751) -> (w750:errorcluster)
          }
        }
        n355 = call-dynamic "Delacor_lib_QMH_Error Handler - Message Handling Loop.vi"("error in"=w276, "Message Queue in"=w266) -> ("dup error in"=w273:errorcluster)  [unwired: 8 in, 1 out]
      }
    }
    frame Error {
      # "Synchronize Caller Events.vi will inform Start Module.vi that the module has launched and will let the code calling Start Module.vi register for broadcasts and would permit the caller receive the broadcast that an error occurred at launch time."
      n356 = call-dynamic "Delacor_lib_QMH_Release Message Queue.vi"("error in"=w762, "Message Queue"=w760) -> ("error out"=w761:errorcluster)  [unwired: 9 in]
      n357 = call "Synchronize Caller Events.vi"("Singleton Module Admin in"=w763) -> ("error out"=w768:errorcluster)  [unwired: 9 in, 1 out]
      n358 = call "Module Name--constant.vi"() -> ("Module Name"=w766:string)  [unwired: 11 in]
      n359 = Format Into String(format string="An error occurred during initialization. %s is no longer running.", w766) -> (resulting string=w764:string)  [unwired: 2 in, 1 out]
      n360 = Merge Errors(w761, w768) -> (w769:errorcluster)
      n361 = call "Error Reported.vi"("Additional Information"=w764, "Error"=w769) -> ()  [unwired: 9 in, 1 out]
    }
  }
  n362 = Merge Errors(w14, w17) -> (w13:errorcluster)
  n363 = call "Close Module.vi"("error in (no error)"=w13, "Module Admin in"=w8) -> ("error out"=w15:errorcluster, "External Launch"=w3:bool, "Module Admin out"=w4:refnum<class "Delacor_lib_QMH_Module Admin.lvclass">)  [unwired: 7 in]
  n364 = Unregister For Events(event registration refnum=w7, error in=w15) -> (error out=w12:errorcluster)
  "error out" <- w12
  n365 = case "External Launch?" shown="True" w3 {
    tunnel: w12 -> [_ w770]
    frame False {
    }
    frame True {
      n366 = case shown="No Error" w770 {
        frame No Error {
          n367 = invoke class="VI" method="FP.Close"() -> ()  [unwired: 3 in, 3 out]
        }
        frame Error {
          n368 = invoke class="VI" method="FP.Open"("Activate"=TRUE ("Activate?")) -> ()  [unwired: 4 in, 5 out]
        }
      }
    }
  }
  n369 = local write "Module Admin"(w4) -> ()
